vi "Read Angel (rad).vi"(11 "ValveModbus in":refnum<class "ValveModbus.lvclass">) -> (2 "Angel (rad)":dbl, 3 "ValveModbus out":refnum<class "ValveModbus.lvclass">)   [LabVIEW 2019, in "ValveModbus.lvclass"]
uses:
  ValveModbus.lvclass
  ValveModbus.lvclass/ValveModbus.ctl
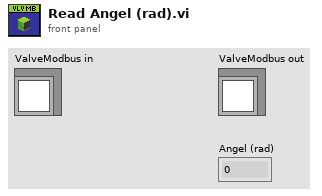
[diagram p1: front panel]
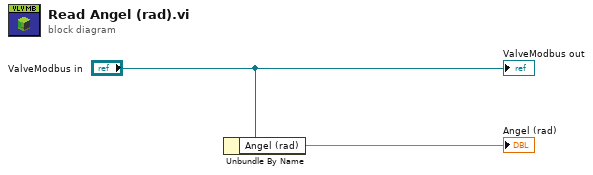
[diagram p0: block diagram]
diagram:
  n1 = Unbundle By Name("ValveModbus in") -> ("Angel (rad)"=→"Angel (rad)":dbl)
  "ValveModbus out" <- "ValveModbus in"
